vi "Demonstrator Main.vi"() -> ()   [LabVIEW 2014]
doc: "This Continuous Measurement sample project is based on the Queued Message Handler template.\n\nThe Event Handling Loop generates messages based on user interface actions.\n\nThe Message Handling Loop processes messages generated by the Event Handling Loop, or by other messages. There are also Acquisition and Logging message handling loop subVIs, and a chart updating loop."
uses:
  Settings/Settings.ctl
  Acquisition/Hardware Configuration.ctl
  Acquisition/Signal Type.ctl
  Logging/Logging Configuration.ctl
  controls/Demonstrator UI Data.ctl
  controls/Demonstrator UI State.ctl
  support/Message Queue/Enqueue Message (Single).vi
  support/Message Queue/Enqueue Message (Array).vi
  <vilib>/Utility/error.llb/Error Cluster From Error Code.vi
  <vilib>/ErrorRing/Error Ring.xnode
  Acquisition/Demonstrator Acquisition.lvlib
  Logging/Demonstrator Logging.lvlib
  Settings/Demonstrator Settings.lvlib
  support/User Event - Stop/Demonstrator User Event - Stop.lvlib
  support/Message Queue/Demonstrator Message Queue.lvlib
panel:
  out "Data":waveform(dbl)[](graph)
  in  "Settings":bool
  in  "Start":bool
  in  "Stop":bool
  out "Status":string
  in  "Exit":bool
  # "Continuous Measurement Data Logger"
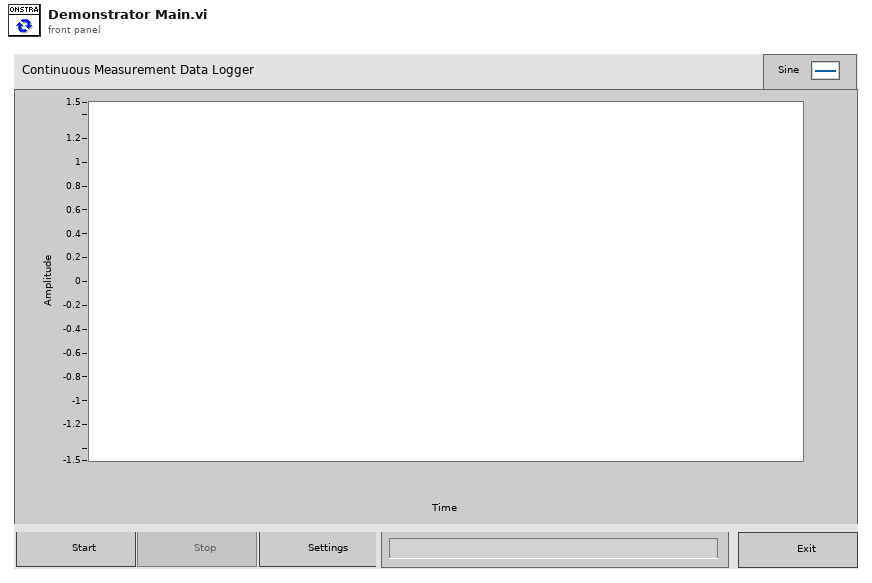
[diagram p1: front panel]
types:
  T1 = typedef "Demonstrator UI State.ctl" = enum16{"Idle", "Acquiring and Logging", "Waiting for Exit", "Waiting for Exit (Acq Stopped)", "Waiting for Exit (Log Stopped)", "Waiting for Stop", "Waiting for Stop (Acq Stopped)", "Waiting for Stop (Log Stopped)"}
  T2 = typedef "Demonstrator UI Data.ctl" = cluster{"Start Ref":refnum<vi>, "Stop Ref":refnum<vi>, "Settings Ref":refnum<vi>, "Exit Ref":refnum<vi>, "Status Ref":refnum<vi>, "Data Ref":refnum<vi>}
  T3 = typedef "Demonstrator Settings.lvlib/Settings.ctl" = cluster{"Hardware Configuration":T4, "Logging Configuration":T6}
  T4 = typedef "Demonstrator Acquisition.lvlib/Hardware Configuration.ctl" = cluster{"HW Refnum <Replace Me>":string, "Signal Type <Replace Me>":T5}
  T5 = typedef "Demonstrator Acquisition.lvlib/Signal Type.ctl" = enum16{"Sine Wave", "Square with Noise"}
  T6 = typedef "Demonstrator Logging.lvlib/Logging Configuration.ctl" = cluster{"Log File Base Path":path, "TDMS File Reference":refnum<k34>}
  T7 = typedef "Demonstrator Message Queue.lvlib/All Message Queues.ctl" = cluster{"UI":refnum<queue>, "Acquisition":refnum<queue>, "Logging":refnum<queue>}
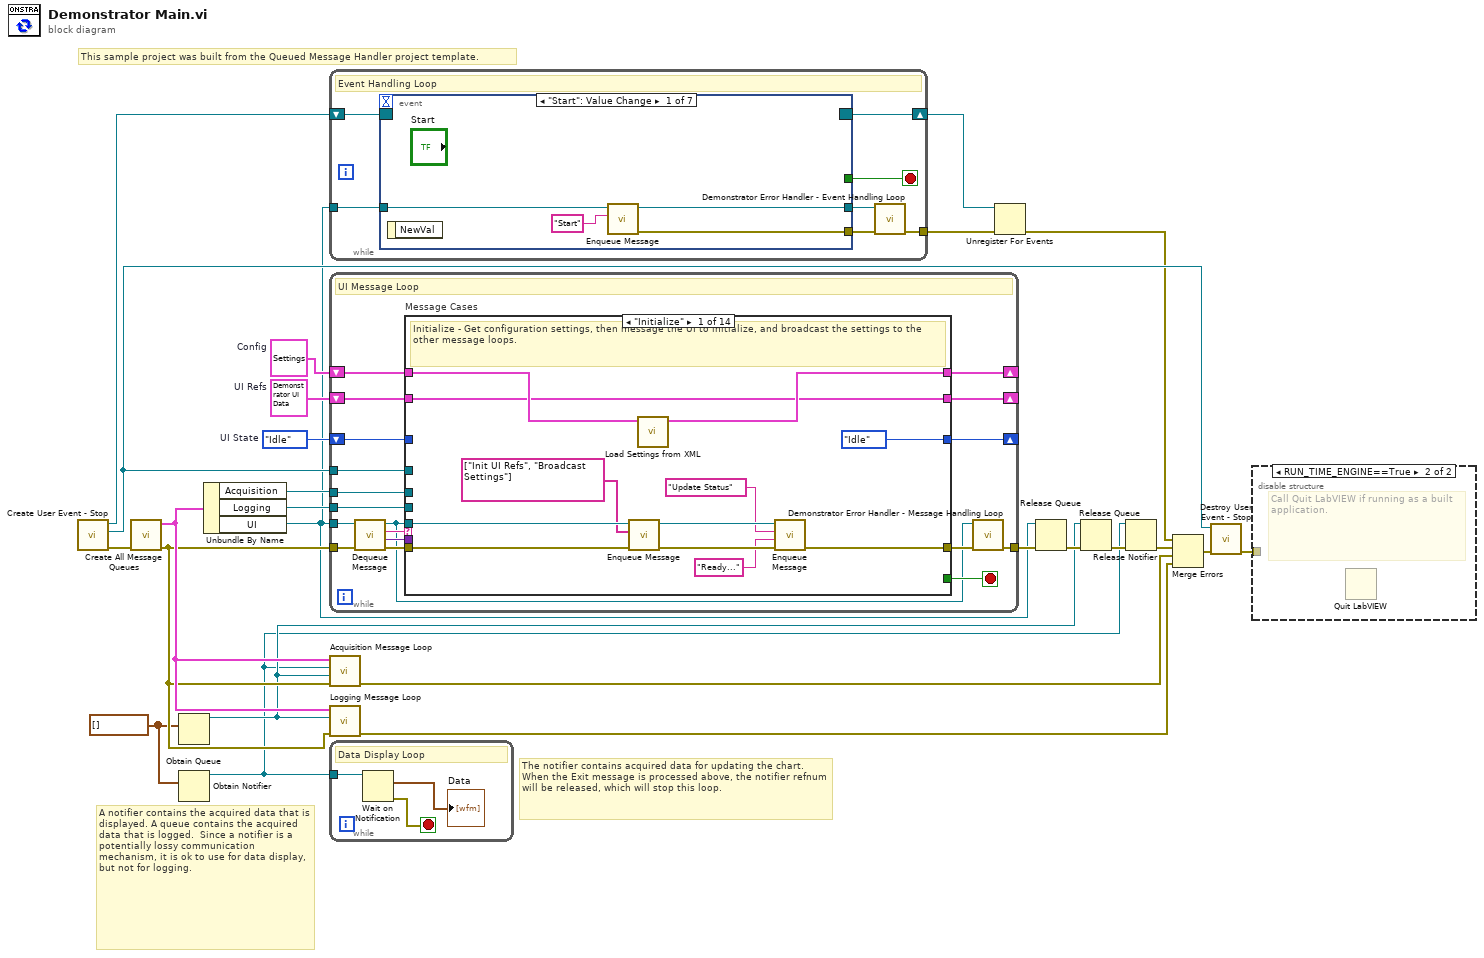
[diagram p0: block diagram]
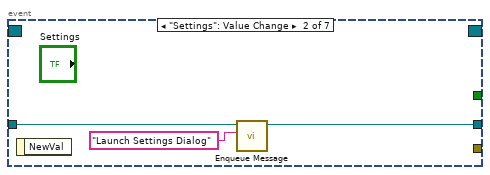
[diagram p3: hidden frame]
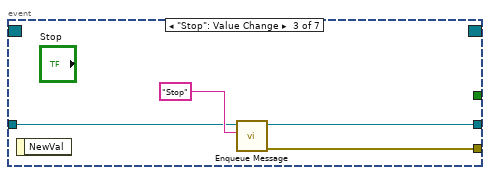
[diagram p4: hidden frame]
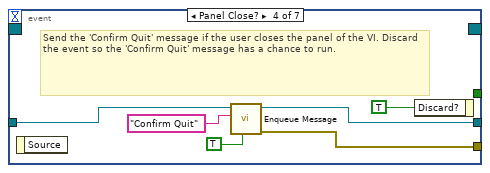
[diagram p5: hidden frame]
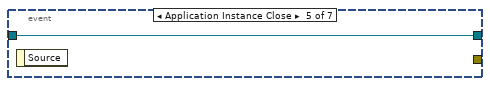
[diagram p6: hidden frame]
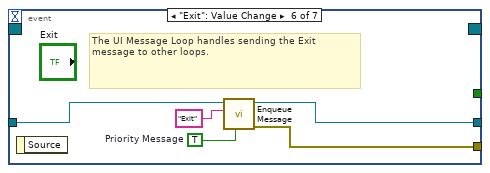
[diagram p7: hidden frame]
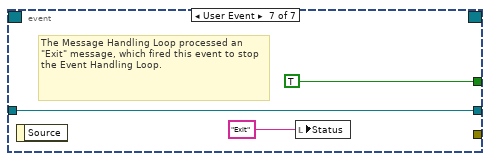
[diagram p8: hidden frame]
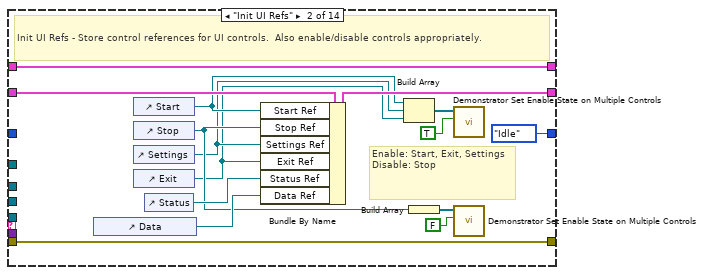
[diagram p9: hidden frame]
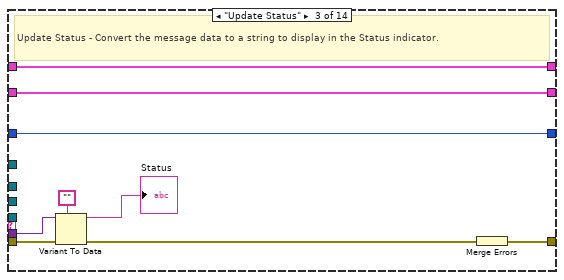
[diagram p10: hidden frame]
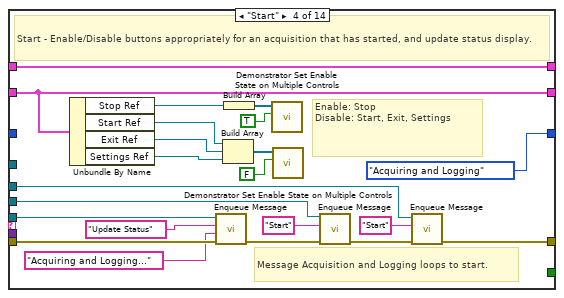
[diagram p11: hidden frame]
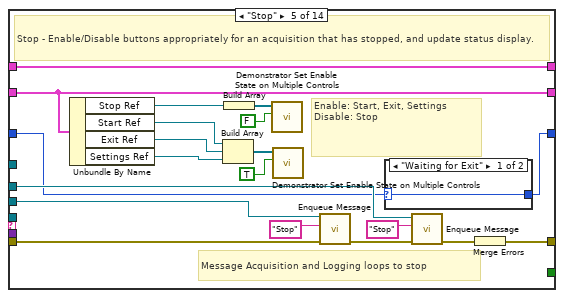
[diagram p12: hidden frame]
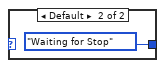
[diagram p13: hidden frame]
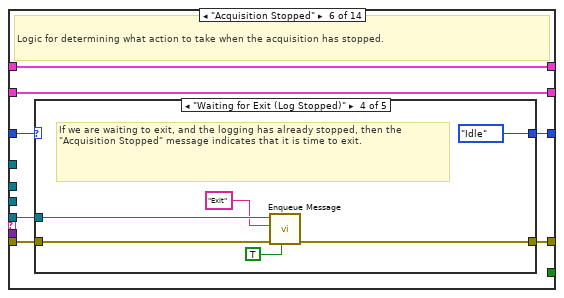
[diagram p14: hidden frame]
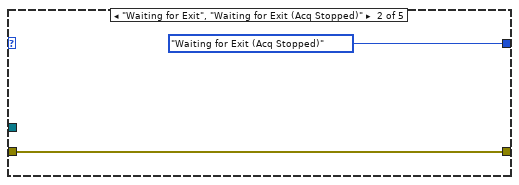
[diagram p16: hidden frame]
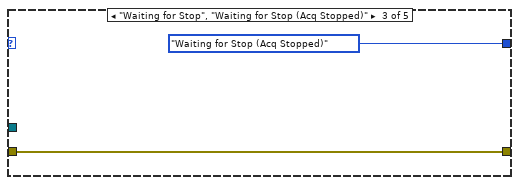
[diagram p17: hidden frame]
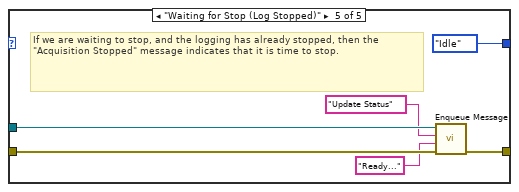
[diagram p18: hidden frame]
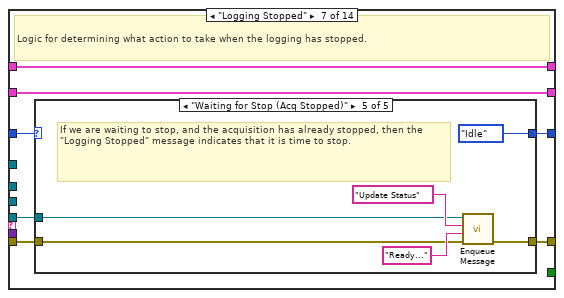
[diagram p19: hidden frame]
diagram:
  w10 = Demonstrator_UI_State."Idle"  # UI State
  w1 = waveform(dbl)[] []
  w13 = T2 {"Start Ref"=refnum, "Stop Ref"=refnum, "Settings Ref"=refnum, "Exit Ref"=refnum, "Status Ref"=refnum, "Data Ref"=refnum}  # UI Refs
  w16 = T3 {"Hardware Configuration"={"HW Refnum <Replace Me>"="", "Signal Type <Replace Me>"=enum."Sine Wave"}, "Logging Configuration"={"Log File Base Path"=path "", "TDMS File Reference"=refnum}}  # Config
  # "This sample project was built from the Queued Message Handler project template."
  # "A notifier contains the acquired data that is displayed. A queue contains the acquired data that is logged.  Since a notifier is a potentially lossy communication mechanism, it is ok to use for data display, but not for logging."
  # "The notifier contains acquired data for updating the chart. When the Exit message is processed above, the notifier refnum will be released, which will stop this loop."
  n1 = call "Create User Event - Stop.vi"() -> ("error out"=w20:errorcluster, "User Event - Stop"=w22:refnum<user-event>, "Stop Event Registration Refnum"=w23:refnum<event-registration>)  [unwired: 9 in]
  n2 = call "Create All Message Queues.vi"("error in (no error)"=w20) -> ("error out"=w17:errorcluster, "Message Queues out"=w19:T7)  [unwired: 9 in]
  n3 = Obtain Queue(element data type=w1) -> (queue out=w3:refnum<queue>)  [unwired: 4 in, 2 out]
  n4 = Obtain Notifier(notification data type=w1) -> (notifier out=w2:refnum<notifier>)  [unwired: 3 in, 2 out]
  n5 = Unbundle By Name(w19) -> ("Acquisition"=w12:refnum<queue>, "Logging"=w11:refnum<queue>, "UI"=w8:refnum<queue>)
  n6 = while {
    tunnel: w8 -> [w31]
    tunnel: [w28] -> w24
    shift-right: [w30] -> w14
    shift-left: w23 -> [w32]
    stop <- w29 stop-if-true
    # "Event Handling Loop"
    n7 = event shown="[0] \"Start\": Value Change" {
      selector: w32 -> [_ _ _ _ _ _ _]
      dyn-events: [_ _ _ _ _ _ _] -> w30
      timeout: _ -> [_ _ _ _ _ _ _]
      tunnel: [_ _ _ _ _ _ TRUE ("Discard?")] -> w29
      tunnel: w31 -> [w36 w38 w42 w47 w50 w52 w56]
      tunnel: [w34 _ w41 w45 _ w55 _] -> w27
      tunnel: [w33 w37 w40 w46 w50 w51 w56] -> w26
      event "Start": Value Change {
        n8 = event-data() -> ()  [unwired: 1 in, 1 out]
        n9 = call-poly "Enqueue Message.vi"("Message"="Start", "Message Queue"=w36) -> ("error out"=w34:errorcluster, "dup Message Queue"=w33:refnum<queue>)  [unwired: 8 in]
      }
      event "Settings": Value Change {
        n10 = event-data() -> ()  [unwired: 1 in, 1 out]
        n11 = call-poly "Enqueue Message.vi"("Message"="Launch Settings Dialog", "Message Queue"=w38) -> ("dup Message Queue"=w37:refnum<queue>)  [unwired: 8 in, 1 out]
      }
      event "Stop": Value Change {
        n12 = event-data() -> ()  [unwired: 1 in, 1 out]
        n13 = call-poly "Enqueue Message.vi"("Message"="Stop", "Message Queue"=w42) -> ("error out"=w41:errorcluster, "dup Message Queue"=w40:refnum<queue>)  [unwired: 8 in]
      }
      event Panel Close? {
        # "Send the 'Confirm Quit' message if the user closes the panel of the VI. Discard the event so the 'Confirm Quit' message has a chance to run."
        n14 = event-data() -> ()  [unwired: 1 in, 1 out]
        n15 = call-poly "Enqueue Message.vi"("Priority Message? (F)"=TRUE, "Message"="Confirm Quit", "Message Queue"=w47) -> ("error out"=w45:errorcluster, "dup Message Queue"=w46:refnum<queue>)  [unwired: 7 in]
        n16 = event-data("Discard?"=TRUE) -> ()  [unwired: 1 in, 1 out]
      }
      event Application Instance Close {
        n17 = event-data() -> ()  [unwired: 1 in, 1 out]
      }
      event "Exit": Value Change {
        w53 = TRUE  # Priority Message
        # "The UI Message Loop handles sending the Exit message to other loops."
        n18 = event-data() -> ()  [unwired: 1 in, 1 out]
        n19 = call-poly "Enqueue Message.vi"("Priority Message? (F)"=w53, "Message"="Exit", "Message Queue"=w52) -> ("error out"=w55:errorcluster, "dup Message Queue"=w51:refnum<queue>)  [unwired: 7 in]
      }
      event User Event {
        # "The Message Handling Loop processed an \"Exit\" message, which fired this event to stop the Event Handling Loop."
        n20 = event-data() -> ()  [unwired: 1 in, 1 out]
        n21 = local write "Status"("Exit" ("Exit String")) -> ()
      }
    }
    n22 = call "Demonstrator Error Handler - Event Handling Loop.vi"("error in (no error)"=w27, "Message Queue"=w26) -> ("dup error in"=w28:errorcluster)  [unwired: 8 in, 1 out]
  }
  n23 = while {
    tunnel: w8 -> [w70]
    tunnel: w22 -> [w75]
    shift-right: [w69] -> _
    shift-left: w16 -> [w68]
    shift-right: [w66] -> _
    shift-left: w13 -> [w67]
    tunnel: w12 -> [w65]
    tunnel: w11 -> [w64]
    shift-right: [w59] -> _
    shift-left: w10 -> [w60]
    tunnel: w17 -> [w74]
    tunnel: [w63] -> w25
    stop <- w76 stop-if-true
    # "UI Message Loop"
    n24 = call "Dequeue Message.vi"("error in (no error)"=w74, "Message Queue"=w70) -> ("error out"=w73:errorcluster, "Message Data"=w71:variant, "Message"=w72:string, "dup Message Queue"=w61:refnum<queue>)  [unwired: 6 in]
    n25 = case "Message Cases" shown="\"Initialize\"" w72 {
      selector: w72 -> [_ _ _ _ _ _ _ _ _ _ _ _ _ w292]
      tunnel: w61 -> [w80 _ _ w134 _ w159 w184 _ w224 w239 w248 _ _ _]
      tunnel: w73 -> [w79 w103 w111 w133 w153 w160 w185 w212 w226 _ w247 w273 w290 _]
      tunnel: [w84 w103 w112 w116 w154 w157 w182 w218 w219 w238 w246 w283 w289 w291] -> w62
      tunnel: [_ _ _ _ _ _ _ _ _ _ _ TRUE _ _] -> w76
      tunnel: w71 -> [_ _ w110 _ _ _ _ _ _ w240 _ _ _ _]
      tunnel: w75 -> [_ _ _ _ _ _ _ _ _ _ _ w284 _ _]
      tunnel: [w87 w102 w106 w132 w152 w163 w188 w216 w223 w244 w251 w282 w288 w295] -> w69
      tunnel: w68 -> [w88 w102 w106 w132 w152 w163 w188 w216 w227 w244 w251 w282 w288 w295]
      tunnel: w67 -> [w81 w101 w105 w129 w151 w162 w187 w210 w221 w243 w250 w281 w287 w294]
      tunnel: [w81 w98 w105 w129 w151 w162 w187 w210 w221 w243 w250 w281 w287 w294] -> w66
      tunnel: w65 -> [_ _ _ w115 w138 _ _ w209 _ _ _ w280 _ _]
      tunnel: w64 -> [_ _ _ w118 w141 _ _ w208 _ _ _ w279 _ _]
      tunnel: w60 -> [_ _ w104 _ w135 w161 w186 w207 w220 w236 w249 _ w286 w293]
      tunnel: [Demonstrator_UI_State."Idle" ("UI State") Demonstrator_UI_State."Idle" ("UI State") w104 Demonstrator_UI_State."Acquiring and Logging" ("UI State") w136 w158 w183 w207 w220 w236 w245 Demonstrator_UI_State."Idle" ("UI State") w286 w293] -> w59
      frame "Initialize" {
        # "Initialize - Get configuration settings, then message the UI to initialize, and broadcast the settings to the other message loops."
        n26 = call-poly "Enqueue Message.vi"("error in (no error)"=w79, "Message Array"=string[] ["Init UI Refs", "Broadcast Settings"], "Message Queue"=w80) -> ("error out"=w86:errorcluster, "dup Message Queue"=w85:refnum<queue>)  [unwired: 7 in]
        n27 = call "Load Settings from XML.vi"("Settings in"=w88) -> ("Settings out"=w87:T3)  [unwired: 9 in, 1 out]
        n28 = call-poly "Enqueue Message.vi"("error in (no error)"=w86, "Message Data"="Ready..." ("Ready..."), "Message"="Update Status", "Message Queue"=w85) -> ("error out"=w84:errorcluster)  [unwired: 6 in, 1 out]
      }
      frame "Init UI Refs" {
        # "Enable: Start, Exit, Settings\nDisable: Stop"
        # "Init UI Refs - Store control references for UI controls.  Also enable/disable controls appropriately."
        n29 = control-ref of="Data"() -> (w99:refnum<vi>)
        n30 = control-ref of="Start"() -> (w92:refnum<vi>)
        n31 = control-ref of="Stop"() -> (w93:refnum<vi>)
        n32 = control-ref of="Settings"() -> (w91:refnum<vi>)
        n33 = control-ref of="Exit"() -> (w90:refnum<vi>)
        n34 = control-ref of="Status"() -> (w100:refnum<vi>)
        n35 = Bundle By Name(cluster=w101, "Start Ref"=w92, "Stop Ref"=w93, "Settings Ref"=w91, "Exit Ref"=w90, "Status Ref"=w100, "Data Ref"=w99) -> (w98:T2)
        n36 = Build Array(w92, w91, w90) -> (w96:refnum<vi>[])
        n37 = Build Array(w93) -> (w95:refnum<vi>[])
        n38 = call "Demonstrator Set Enable State on Multiple Controls.vi"("Enable?"=TRUE, "Controls"=w96) -> ()  [unwired: 10 in]
        n39 = call "Demonstrator Set Enable State on Multiple Controls.vi"("Enable?"=FALSE, "Controls"=w95) -> ()  [unwired: 10 in]
      }
      frame "Update Status" {
        # "Update Status - Convert the message data to a string to display in the Status indicator."
        n40 = Variant To Data(error in=w111, type="", Variant=w110) -> (data=→"Status":string, error out=w108:errorcluster)
        n41 = Merge Errors(w108) -> (w112:errorcluster)
      }
      frame "Start" {
        # "Message Acquisition and Logging loops to start."
        # "Enable: Stop\nDisable: Start, Exit, Settings"
        # "Start - Enable/Disable buttons appropriately for an acquisition that has started, and update status display."
        n42 = Unbundle By Name(w129) -> ("Stop Ref"=w124:refnum<vi>, "Start Ref"=w123:refnum<vi>, "Exit Ref"=w122:refnum<vi>, "Settings Ref"=w121:refnum<vi>)
        n43 = call-poly "Enqueue Message.vi"("error in (no error)"=w133, "Message Data"="Acquiring and Logging..." ("Acquiring and Logging..."), "Message"="Update Status", "Message Queue"=w134) -> ("error out"=w120:errorcluster)  [unwired: 6 in, 1 out]
        n44 = Build Array(w123, w122, w121) -> (w127:refnum<vi>[])
        n45 = Build Array(w124) -> (w126:refnum<vi>[])
        n46 = call "Demonstrator Set Enable State on Multiple Controls.vi"("Enable?"=TRUE, "Controls"=w126) -> ()  [unwired: 10 in]
        n47 = call "Demonstrator Set Enable State on Multiple Controls.vi"("Enable?"=FALSE, "Controls"=w127) -> ()  [unwired: 10 in]
        n48 = call-poly "Enqueue Message.vi"("error in (no error)"=w120, "Message"="Start", "Message Queue"=w118) -> ("error out"=w117:errorcluster)  [unwired: 7 in, 1 out]
        n49 = call-poly "Enqueue Message.vi"("error in (no error)"=w117, "Message"="Start", "Message Queue"=w115) -> ("error out"=w116:errorcluster)  [unwired: 7 in, 1 out]
      }
      frame "Stop" {
        # "Message Acquisition and Logging loops to stop"
        # "Enable: Start, Exit, Settings\nDisable: Stop"
        # "Stop - Enable/Disable buttons appropriately for an acquisition that has stopped, and update status display."
        n50 = Unbundle By Name(w151) -> ("Stop Ref"=w146:refnum<vi>, "Start Ref"=w145:refnum<vi>, "Exit Ref"=w144:refnum<vi>, "Settings Ref"=w143:refnum<vi>)
        n51 = Build Array(w145, w144, w143) -> (w149:refnum<vi>[])
        n52 = Build Array(w146) -> (w148:refnum<vi>[])
        n53 = call "Demonstrator Set Enable State on Multiple Controls.vi"("Enable?"=FALSE, "Controls"=w148) -> ()  [unwired: 10 in]
        n54 = call "Demonstrator Set Enable State on Multiple Controls.vi"("Enable?"=TRUE, "Controls"=w149) -> ()  [unwired: 10 in]
        n55 = call-poly "Enqueue Message.vi"("error in (no error)"=w153, "Message"="Stop", "Message Queue"=w141) -> ("error out"=w140:errorcluster)  [unwired: 7 in, 1 out]
        n56 = case shown="\"Waiting for Exit\"" w135 {
          selector: w135 -> [w155 _]
          tunnel: [w155 Demonstrator_UI_State."Waiting for Stop" ("UI State")] -> w136
          frame "Waiting for Exit" {
          }
          frame Default {
          }
        }
        n57 = call-poly "Enqueue Message.vi"("error in (no error)"=w140, "Message"="Stop", "Message Queue"=w138) -> ("error out"=w139:errorcluster)  [unwired: 7 in, 1 out]
        n58 = Merge Errors(w139) -> (w154:errorcluster)
      }
      frame "Acquisition Stopped" {
        # "Logic for determining what action to take when the acquisition has stopped."
        n59 = case shown="\"Waiting for Exit (Log Stopped)\"" w161 {
          selector: w161 -> [w165 _ _ _ _]
          tunnel: w160 -> [w164 w167 w169 w175 w181]
          tunnel: w159 -> [_ _ _ w173 w178]
          tunnel: [w165 Demonstrator_UI_State."Waiting for Exit (Acq Stopped)" ("UI State") Demonstrator_UI_State."Waiting for Stop (Acq Stopped)" ("UI State") Demonstrator_UI_State."Idle" ("UI State") Demonstrator_UI_State."Idle" ("UI State")] -> w158
          tunnel: [w164 w167 w169 w174 w179] -> w157
          frame Default {
          }
          frame "Waiting for Exit", "Waiting for Exit (Acq Stopped)" {
          }
          frame "Waiting for Stop", "Waiting for Stop (Acq Stopped)" {
          }
          frame "Waiting for Exit (Log Stopped)" {
            # "If we are waiting to exit, and the logging has already stopped, then the \"Acquisition Stopped\" message indicates that it is time to exit."
            n60 = call-poly "Enqueue Message.vi"("Priority Message? (F)"=TRUE, "error in (no error)"=w175, "Message"="Exit", "Message Queue"=w173) -> ("error out"=w174:errorcluster)  [unwired: 6 in, 1 out]
          }
          frame "Waiting for Stop (Log Stopped)" {
            # "If we are waiting to stop, and the logging has already stopped, then the \"Acquisition Stopped\" message indicates that it is time to stop."
            n61 = call-poly "Enqueue Message.vi"("error in (no error)"=w181, "Message Data"="Ready..." ("Ready..."), "Message"="Update Status", "Message Queue"=w178) -> ("error out"=w179:errorcluster)  [unwired: 6 in, 1 out]
          }
        }
      }
      frame "Logging Stopped" {
        # "Logic for determining what action to take when the logging has stopped."
        n62 = case shown="\"Waiting for Stop (Acq Stopped)\"" w186 {
          selector: w186 -> [w190 _ _ _ _]
          tunnel: w185 -> [w189 w192 w194 w200 w203]
          tunnel: w184 -> [_ _ _ w198 w202]
          tunnel: [w190 Demonstrator_UI_State."Waiting for Exit (Log Stopped)" ("UI State") Demonstrator_UI_State."Waiting for Stop (Log Stopped)" ("UI State") Demonstrator_UI_State."Idle" ("UI State") Demonstrator_UI_State."Idle" ("UI State")] -> w183
          tunnel: [w189 w192 w194 w199 w201] -> w182
          frame Default {
          }
          frame "Waiting for Exit", "Waiting for Exit (Log Stopped)" {
          }
          frame "Waiting for Stop", "Waiting for Stop (Log Stopped)" {
          }
          frame "Waiting for Exit (Acq Stopped)" {
            # "If we are waiting to exit, and the acquisition has already stopped, then the \"Logging Stopped\" message indicates that it is time to exit."
            n63 = call-poly "Enqueue Message.vi"("Priority Message? (F)"=TRUE, "error in (no error)"=w200, "Message"="Exit", "Message Queue"=w198) -> ("error out"=w199:errorcluster)  [unwired: 6 in, 1 out]
          }
          frame "Waiting for Stop (Acq Stopped)" {
            # "If we are waiting to stop, and the acquisition has already stopped, then the \"Logging Stopped\" message indicates that it is time to stop."
            n64 = call-poly "Enqueue Message.vi"("error in (no error)"=w203, "Message Data"="Ready..." ("Ready..."), "Message"="Update Status", "Message Queue"=w202) -> ("error out"=w201:errorcluster)  [unwired: 6 in, 1 out]
          }
        }
      }
      frame "Broadcast settings" {
        w211 = "Update Settings" ("Message")
        # "Broadcast settings - Send the 'Update Settings' message to the Logging and Acquisition message loops."
        n65 = Unbundle By Name(w216) -> ("Hardware Configuration"=w215:T4, "Logging Configuration"=w214:T6)
        n66 = call-poly "Enqueue Message.vi"("Message Data"=w215, "Message"=w211, "Message Queue"=w209) -> ("error out"=w217:errorcluster)  [unwired: 7 in, 1 out]
        n67 = call-poly "Enqueue Message.vi"("error in (no error)"=w217, "Message Data"=w214, "Message"=w211, "Message Queue"=w208) -> ("error out"=w213:errorcluster)  [unwired: 6 in, 1 out]
        n68 = Merge Errors(w213, w212) -> (w218:errorcluster)
      }
      frame "Launch Settings Dialog" {
        # "Launch Settings Dialog - Launch the Settings Dialog when the user clicks the 'Settings' button."
        n69 = call "Settings Dialog.vi"("error in (no error)"=w226, "Settings in"=w227) -> ("error out"=w222:errorcluster, "Cancelled?"=w225:bool, "Settings out"=w223:T3)  [unwired: 6 in, 1 out]
        n70 = case shown="False" w225 {
          tunnel: w224 -> [w231 _]
          tunnel: w222 -> [w230 w232]
          tunnel: [w229 w232] -> w219
          frame False {
            n71 = call-poly "Enqueue Message.vi"("error in (no error)"=w230, "Message"="Broadcast Settings", "Message Queue"=w231) -> ("error out"=w229:errorcluster)  [unwired: 7 in, 1 out]
          }
          frame True {
          }
        }
      }
      frame "Error" {
        # "Always cast error data, even on incoming error."
        # "Error - Check the error message data and respond accordingly. This message is sent by the \"Error Handler\" VIs at the end of each loop in this application."
        n72 = Variant To Data(type=errorcluster {"status"=FALSE, "code"=0, "source"=""} ("error constant"), Variant=w240) -> (data=w235:errorcluster, error out=w241:errorcluster)  [unwired: 1 in]
        n73 = call <vilib>:"Simple Error Handler.vi"("error in (no error)"=w235) -> ()  [unwired: 4 in, 5 out]
        n74 = call-poly "Enqueue Message.vi"("Priority Message? (F)"=TRUE, "Message"="Exit", "Message Queue"=w239) -> ("error out"=w237:errorcluster)  [unwired: 7 in, 1 out]
        n75 = Merge Errors(w237, w241) -> (w238:errorcluster)
      }
      frame "Confirm Quit" {
        # "Confirm Quit - Message that can confirm whether or not the user wants to exit the application."
        n76 = case shown="\"Acquiring and Logging\"" w249 {
          tunnel: w248 -> [w257 w261]
          tunnel: w247 -> [w256 w260]
          tunnel: [w255 w259] -> w246
          tunnel: [Demonstrator_UI_State."Idle" ("UI State") w258] -> w245
          frame Default {
            # "If 'Confirm Quit' comes in while the system is idle, there is no need for a confirmation message."
            n77 = call-poly "Enqueue Message.vi"("Priority Message? (F)"=TRUE, "error in (no error)"=w256, "Message"="Exit", "Message Queue"=w257) -> ("error out"=w255:errorcluster)  [unwired: 6 in, 1 out]
          }
          frame "Acquiring and Logging" {
            n78 = Two Button Dialog(message="Are you sure you want to quit while the acquisition is running?" ("Confirm Quit Message"), 1:"No" ("No"), 2:"Yes" ("Yes")) -> (T button?=w262:bool)
            n79 = case shown="True" w262 {
              tunnel: w261 -> [_ w271]
              tunnel: w260 -> [w267 w272]
              tunnel: [w267 w270] -> w259
              tunnel: [Demonstrator_UI_State."Acquiring and Logging" ("UI State") Demonstrator_UI_State."Waiting for Exit" ("UI State")] -> w258
              frame False {
                # "User did not want to quit."
              }
              frame True {
                n80 = call-poly "Enqueue Message.vi"("error in (no error)"=w272, "Message"="Stop", "Message Queue"=w271) -> ("error out"=w270:errorcluster)  [unwired: 7 in, 1 out]
              }
            }
          }
        }
      }
      frame "Exit" {
        w275 = TRUE ("Priority Message? (F)")
        w276 = "Exit" ("Message")
        # "Stop the VI"
        # "Exit - Send Exit messages to the Acquisition and Logging loops, and fire the user event to stop the Event Handling Loop."
        n81 = call-poly "Enqueue Message.vi"("Priority Message? (F)"=w275, "error in (no error)"=w273, "Message"=w276, "Message Queue"=w280) -> ("error out"=w277:errorcluster)  [unwired: 6 in, 1 out]
        n82 = call-poly "Enqueue Message.vi"("Priority Message? (F)"=w275, "error in (no error)"=w277, "Message"=w276, "Message Queue"=w279) -> ("error out"=w274:errorcluster)  [unwired: 6 in, 1 out]
        n83 = call "Fire User Event - Stop.vi"("error in (no error)"=w274, "User Event - Stop"=w284) -> ("error out"=w283:errorcluster)  [unwired: 9 in]
      }
      frame "---Copy This Frame---" {
        # "Duplicate this frame when creating new messages.  Change this comment in the duplicated frame to describe this message."
        n84 = Merge Errors(w290) -> (w289:errorcluster)
      }
      frame Default {
        # "'Default' case only runs if there is a message that isn't defined in any of the other cases.  Output a programming error."
        n85 = xnode "Error Ring"("parameter 0"=w292) -> ("error out"=w291:errorcluster)
      }
    }
    n86 = call "Demonstrator Error Handler - Message Handling Loop.vi"("error in (no error)"=w62, "Message Queue"=w61) -> ("dup error in"=w63:errorcluster)  [unwired: 8 in, 1 out]
  }
  n87 = call "Acquisition Message Loop.vi"("error in (no error)"=w17, "Data Queue"=w3, "Data Notifier"=w2, "Message Queues"=w19) -> ("error out"=w21:errorcluster)  [unwired: 7 in]
  n88 = call "Logging Message Loop.vi"("error in (no error)"=w17, "Data Queue"=w3, "Message Queues"=w19) -> ("error out"=w18:errorcluster)  [unwired: 8 in]
  n89 = while "Data Display Loop" {
    tunnel: w2 -> [w305]
    stop <- w303 stop-if-true
    # "Data Display Loop"
    n90 = Wait on Notification(notifier=w305) -> (notification=→"Data":waveform(dbl)[], error out=w303:errorcluster)  [unwired: 3 in, 2 out]
  }
  n91 = Unregister For Events(event registration refnum=w14, error in=w24) -> (error out=w15:errorcluster)
  n92 = Release Queue(queue=w8, error in (no error)=w25) -> (error out=w6:errorcluster)  [unwired: 1 in, 2 out]
  n93 = Release Queue(queue=w3, error in (no error)=w6) -> (error out=w5:errorcluster)  [unwired: 1 in, 2 out]
  n94 = Release Notifier(notifier=w2, error in (no error)=w5) -> (error out=w4:errorcluster)  [unwired: 1 in, 2 out]
  n95 = Merge Errors(w15, w4, w21, w18) -> (w9:errorcluster)
  n96 = call "Destroy User Event - Stop.vi"("error in (no error)"=w9, "User Event - Stop"=w22) -> ("error out"=w7:errorcluster)  [unwired: 9 in]
  n97 = disable-structure shown="RUN_TIME_ENGINE==True" {
    disable-tunnel: w7 -> [_ _]
    frame condition #0 (active) {
    }
    frame condition #1 {
      # "Call Quit LabVIEW if running as a built application."
      n98 = Quit LabVIEW() -> ()  [unwired: 1 in]
    }
  }
